vi "Read 8 Input Logic Operation Result.vi"(7 "Unit Address (1)":u8=1, 8 "error in (no error)":errorcluster, 10 "Selected Function (1)":u8=1 min=1 max=24, 11 "VISA resource name":refnum<visa-resource-name>) -> (0 "error out":errorcluster, 2 "Result":bool, 3 "VISA resource name out":refnum<visa-resource-name>)   [LabVIEW 2014, in "Eurotherm 35xx Series.lvlib"]
doc: "This VI reads the output value of the 8 input logic operation function."
uses:
  <instrlib>/Eurotherm 35xx Series/Eurotherm 35xx Series.lvlib
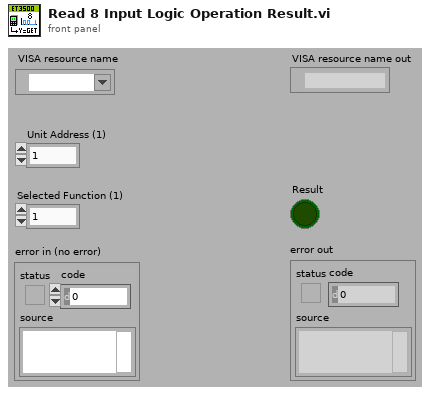
[diagram p1: front panel]
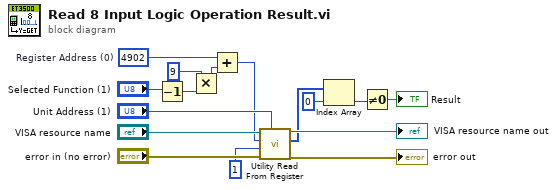
[diagram p0: block diagram]
diagram:
  w5 = 4902  # Register Address (0)
  n1 = Decrement(x="Selected Function (1)") -> (x-1=w10:u8)
  n2 = Multiply(x=u8 9, y=w10) -> (x*y=w8:u8)
  n3 = Add(x=w5, y=w8) -> (x+y=w6:i32)
  n4 = call <instrlib>:"Utility Read From Register.vi"("Unit Address (1)"="Unit Address (1)", "error in (no error)"="error in (no error)", "Num Of Reg (1)"=u16 1, "Register Address (0)"=w6, "VISA resource name"="VISA resource name") -> ("error out"=→"error out":errorcluster, "Data"=w4:i16[], "VISA resource name out"=→"VISA resource name out":refnum<visa-resource-name>)  [unwired: 4 in]
  n5 = Index Array(array=w4, index=0) -> (element=w2:i16)
  n6 = Not Equal To 0?(x=w2) -> (x != 0?=→"Result":bool)
